vi "SM_TEST_A.vi"() -> ()   [LabVIEW 2021]
uses:
  <vilib>/measure/NI_MABase.lvlib
panel:
  out "Waveform Graph":waveform(dbl)(graph)
  in  "phase":dbl
  in  "offset":dbl
  in  "amplitude":dbl
  in  "time scale":dbl
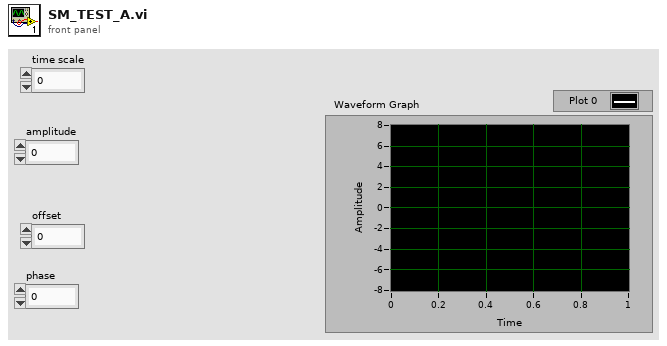
[diagram p1: front panel]
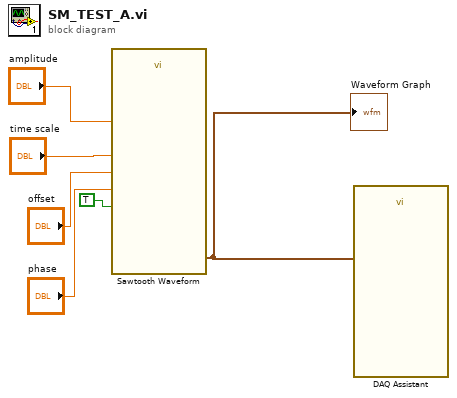
[diagram p0: block diagram]
diagram:
  n1 = call <vilib>:"Sawtooth Waveform.vi"("offset"="offset", "reset signal"=TRUE, "phase"="phase", "amplitude"="amplitude", "frequency"="time scale") -> ("signal out"=w2:waveform(dbl))  [unwired: 5 in, 1 out]
  "Waveform Graph" <- w2
  n2 = call "DAQ Assistant"("data"=w2) -> ()  [unwired: 17 in, 2 out]
